vi "DrivePathToTarget-C.vi"() -> ()   [LabVIEW 2018]
uses:
  Dawgma Programming Library/Controls/PurePursuit/RobotNeededPathData.ctl
  Framework/Robot Global Data.vi
  Drive/Implementation/Drive Published Globals.vi
panel:
  in  "Params":string[][](array[string])
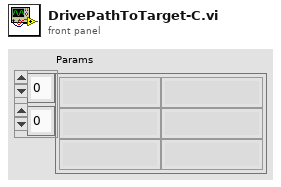
[diagram p1: front panel]
types:
  T1 = typedef "RobotNeededPathData.ctl" = cluster{"Path":cluster{dbl, dbl}[], "MaxVel":dbl, "MaxAccel":dbl, "Backwards?":bool, "PointSpacing":dbl, "LookaheadDist":dbl, "Speed/Curve":dbl, "SlowDistanceAtEnd":dbl, "SlowSpeed":dbl, "MaxDeAccel":dbl}
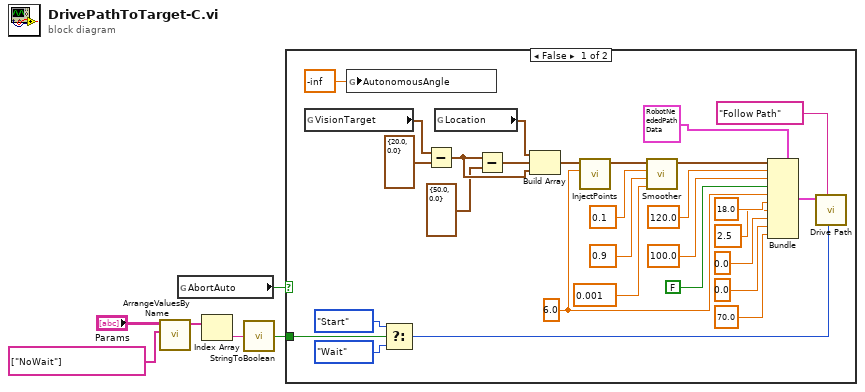
[diagram p0: block diagram]
diagram:
  n1 = call "ArrangeValuesByName.vi"("Names"=string[] ["NoWait"], "Names/Values in"="Params") -> ("Values Out"=w2:string[])  [unwired: 9 in]
  n2 = global read "Robot Global Data.vi" "AbortAuto"() -> (w6:bool)
  n3 = Index Array(array=w2) -> (element=w1:string)  [unwired: 1 in]
  n4 = call "StringToBoolean.vi"("String"=w1) -> ("Output"=w5:bool)
  n5 = case shown="False" w6 {
    tunnel: w5 -> [w7 _]
    frame False {
      w21 = 6.0 ("Distance")
      n6 = global read "Robot Global Data.vi" "VisionTarget"() -> (w34:cluster{"X":dbl, "Y":dbl})
      n7 = global write "Robot Global Data.vi" "AutonomousAngle"(-inf ("AutonomousAngle")) -> ()
      n8 = Select(t=enum16{"Start", "Wait"}."Start" ("Synchronication"), s=w7, f=enum16{"Start", "Wait"}."Wait") -> (s? t:f=w8:enum16{"Start", "Wait"})
      n9 = Subtract(x=w34, y=cluster{dbl, dbl} {20.0, 0.0}) -> (x-y=w33:cluster{dbl, dbl})
      n10 = global read "Drive Published Globals.vi" "Location"() -> (w31:cluster{dbl, dbl})
      n11 = Subtract(x=w33, y=cluster{dbl, dbl} {50.0, 0.0}) -> (x-y=w32:cluster{dbl, dbl})
      n12 = Build Array(w31, w32, w33) -> (w11:cluster{dbl, dbl}[])
      n13 = call "InjectPoints.vi"("Spacing"=w21, "Path"=w11) -> ("Path out"=w27:cluster{dbl, dbl}[])  [unwired: 9 in]
      n14 = call "Smoother.vi"("tolerance"=0.001, "B"=0.9, "A"=0.1, "Path"=w27) -> ("SmoothPath"=w28:cluster{dbl, dbl}[])  [unwired: 7 in]
      n15 = Bundle(cluster=T1 {"Path"=[], "MaxVel"=0.0, "MaxAccel"=0.0, "Backwards?"=FALSE, "PointSpacing"=0.0, "LookaheadDist"=0.0, "Speed/Curve"=1.8, "SlowDistanceAtEnd"=12.0, "SlowSpeed"=15.0, "MaxDeAccel"=0.0} ("Path"), "Path"=w28, "MaxVel"=120.0, "MaxAccel"=100.0, "Backwards?"=FALSE, "PointSpacing"=w21, "LookaheadDist"=18.0, "Speed/Curve"=2.5, "SlowDistanceAtEnd"=0.0, "SlowSpeed"=0.0, "MaxDeAccel"=70.0) -> (w26:T1)
      n16 = call "Drive Path.vi"("Synchronication"=w8, "Description"="Follow Path", "Path"=w26) -> ()  [unwired: 8 in, 1 out]
    }
    frame True {
    }
  }
